vi "Browse.vi"(8 "error in (no error)":errorcluster, 11 "Dynamic Combobox in":refnum<class "Dynamic Combobox.lvclass">) -> (0 "error out":errorcluster, 1 "Cancelled?":bool, 2 "Selected Value":string, 3 "Dynamic Combobox out":refnum<class "Dynamic Combobox.lvclass">)   [LabVIEW 2020, in "Dynamic Combobox.lvlib" / "Dynamic Combobox.lvclass"]
uses:
  Dynamic Combobox.lvclass
  Dynamic Combobox.lvclass/Dynamic Combobox.ctl
  Dynamic Values/Dynamic Values.lvclass
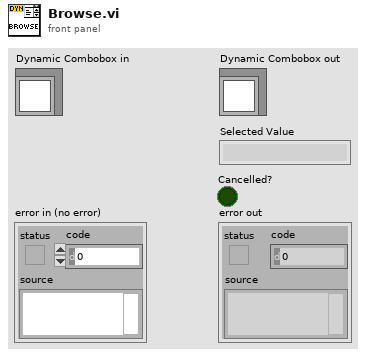
[diagram p1: front panel]
types:
  T1 = typedef "Dynamic Combobox.lvlib/Dynamic Combobox.lvclass/Ref Data.ctl" = cluster{"Values":refnum<class "Dynamic Values.lvclass">, "Debug":bool, "Strings And Values []":T2, "Options":T3}
  T2 = typedef "LVComboBoxStrsAndValuesArrayTypeDef.ctl" = cluster{"String":string, "Value":string}[]
  T3 = typedef "Dynamic Combobox.lvlib/Dynamic Combobox.lvclass/Options.ctl" = cluster{"Browse Entry":bool, "Refresh Entry":bool, "Allow Undefined Values":bool}
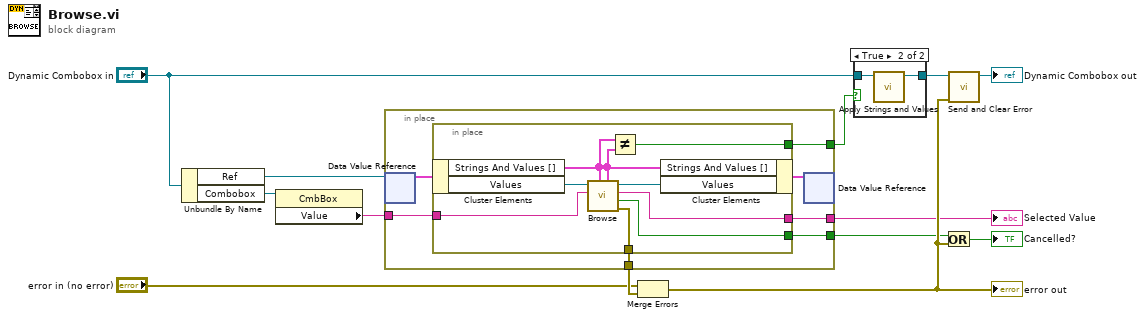
[diagram p0: block diagram]
diagram:
  n1 = Unbundle By Name("Dynamic Combobox in") -> ("Ref"=w11:refnum<data-value>, "Combobox"=w12:refnum<vi>)
  n2 = property class="CmbBox"(reference=w12) -> ("Value"=w10:string)  [unwired: 1 in, 2 out]
  n3 = in-place {
    in-place-border: w10 -> [w15]
    in-place-border: [w19] -> w9
    in-place-border: [w18] -> w5
    in-place-border: [w16] -> w8
    in-place-border: [w14] -> w1
    n4 = in-place-dvr #1(w11) -> (w20:T1)  [unwired: 1 out]
    n5 = in-place {
      in-place-border: [w27] -> w19
      in-place-border: [w26] -> w18
      in-place-border: [w25] -> w16
      in-place-border: w15 -> [w24]
      in-place-border: [w21] -> w14
      n6 = in-place-cluster #2(w20) -> ("Strings And Values []"=w22:T2, "Values"=w29:refnum<class "Dynamic Values.lvclass">)
      n7 = call-dynamic "Browse.vi"("Current Strings and Values"=w22, "Current Value"=w24, "Dynamic Values in"=w29) -> ("error out"=w25:errorcluster, "Cancelled?"=w26:bool, "Selected Value"=w27:string, "Dynamic Values out"=w28:refnum<class "Dynamic Values.lvclass">, "Strings and Values []"=w23:T2)  [unwired: 4 in]
      n8 = Not Equal?(x=w22, y=w23) -> (x != y?=w21:bool)
      n9 = in-place-cluster #2("Strings And Values []"=w23, "Values"=w28) -> (w17:T1)
    }
    n10 = in-place-dvr #1(w17) -> ()  [unwired: 2 out]
  }
  "Selected Value" <- w9
  n11 = Merge Errors("error in (no error)", w8) -> (w13:errorcluster)
  "error out" <- w13
  n12 = case shown="True" w1 {
    tunnel: [w30 w32] -> w3
    tunnel: "Dynamic Combobox in" -> [w30 w31]
    frame False {
    }
    frame True {
      n13 = call "Apply Strings and Values.vi"("Dynamic Combobox in"=w31) -> ("Dynamic Combobox out"=w32:refnum<class "Dynamic Combobox.lvclass">)  [unwired: 9 in, 1 out]
    }
  }
  n14 = Or(x=w5, y=w13) -> (x .or. y?=→"Cancelled?":bool)
  n15 = call "Send and Clear Error.vi"("error in (no error)"=w13, "Dynamic Combobox in"=w3) -> ("Dynamic Combobox out"=→"Dynamic Combobox out":refnum<class "Dynamic Combobox.lvclass">)  [unwired: 8 in, 1 out]
